vi "Write with header.vi"() -> ()   [LabVIEW 2022 SP3]
uses:
  <vilib>/Utility/file.llb/Write Delimited Spreadsheet (string).vi
  <vilib>/Utility/file.llb/Write Delimited Spreadsheet (DBL).vi
panel:
  in  "stop":bool
  out "appended array":dbl[][](array[numeric])
  in  "file path (dialog if empty)":path
  out "Array":string[](array[string])
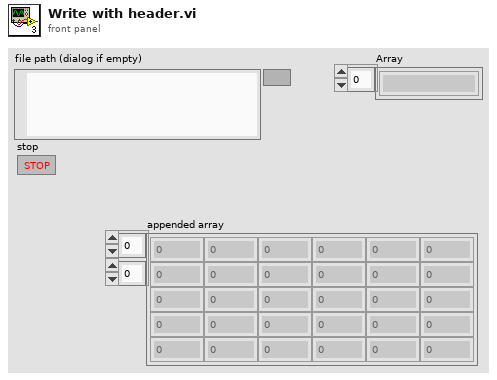
[diagram p1: front panel]
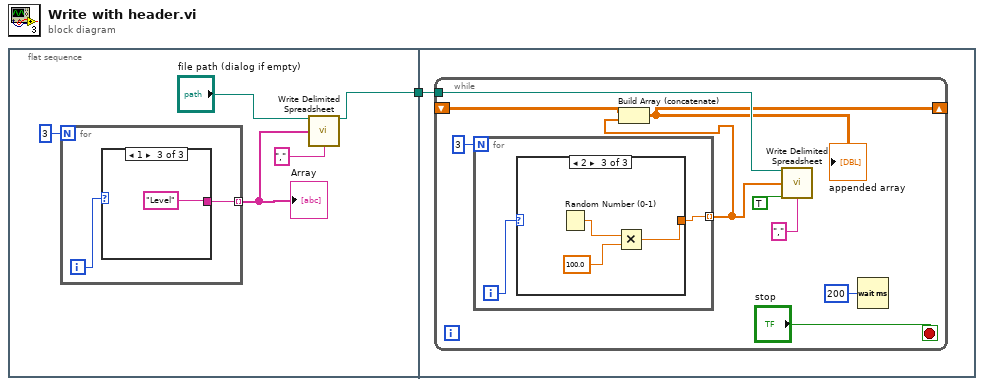
[diagram p0: block diagram]
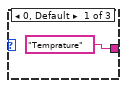
[diagram p2: hidden frame]
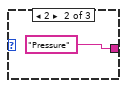
[diagram p3: hidden frame]
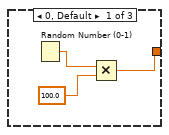
[diagram p4: hidden frame]
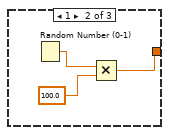
[diagram p5: hidden frame]
diagram:
  n1 = flat-sequence {
    tunnel: [w2] -> w1
    tunnel: w1 -> [w12]
    frame #0 {
      n2 = for {
        N: 3 -> [_]
        tunnel: [w7] -> w3 mode=indexing
        i -> [w8]
        n3 = case shown="1" w8 {
          tunnel: ["Temprature" "Pressure" "Level"] -> w7
          frame 0, Default {
          }
          frame 2 {
          }
          frame 1 {
          }
        }
      }
      "Array" <- w3
      n4 = call-poly <vilib>:"Write Delimited Spreadsheet.vi"("file path (dialog if empty)"="file path (dialog if empty)", "1D data"=w3, "delimiter (\\t)"="," ("delimiter (\\t)")) -> ("new file path (Not A Path if cancelled)"=w2:path)  [unwired: 11 in, 1 out]
    }
    frame #1 {
      n5 = while {
        tunnel: w12 -> [w18]
        shift-right: [w14] -> _
        shift-left: _ -> [w15]
        stop <- "stop" stop-if-true
        n6 = for {
          N: 3 -> [_]
          tunnel: [w22] -> w16 mode=indexing
          i -> [w23]
          n7 = case shown="2" w23 {
            tunnel: [w24 w27 w30] -> w22
            frame 0, Default {
              n8 = Random Number (0-1)() -> (number: 0 to 1=w26:dbl)
              n9 = Multiply(x=w26, y=100.0) -> (x*y=w24:dbl)
            }
            frame 1 {
              n10 = Random Number (0-1)() -> (number: 0 to 1=w29:dbl)
              n11 = Multiply(x=w29, y=100.0) -> (x*y=w27:dbl)
            }
            frame 2 {
              n12 = Random Number (0-1)() -> (number: 0 to 1=w32:dbl)
              n13 = Multiply(x=w32, y=100.0) -> (x*y=w30:dbl)
            }
          }
        }
        n14 = Build Array (concatenate)(w15, w16) -> (w14:dbl[][])
        "appended array" <- w14
        n15 = call-poly <vilib>:"Write Delimited Spreadsheet.vi"("file path (dialog if empty)"=w18, "1D data"=w16, "append to file? (new file:F)"=TRUE, "delimiter (\\t)"="," ("delimiter (\\t)")) -> ()  [unwired: 10 in, 2 out]
        n16 = Wait (ms)(milliseconds to wait=u32 200) -> ()  [unwired: 1 out]
      }
    }
  }
